vi "Create True Constant.vi"(5 "Sink":refnum<vi>, 6 "relative position/next to refnum":T1, 8 "error in (no error)":errorcluster, 11 "Diagram":refnum<vi>) -> (0 "error out":errorcluster, 2 "Output Terminal":refnum<vi>, 3 "constant out":refnum<vi>)   [LabVIEW 2018, in "Scripting Tools.lvlib"]
uses:
  Scripting Tools.lvlib
  <vilib>/Utility/miscctls.llb/LVPointTypeDef.ctl
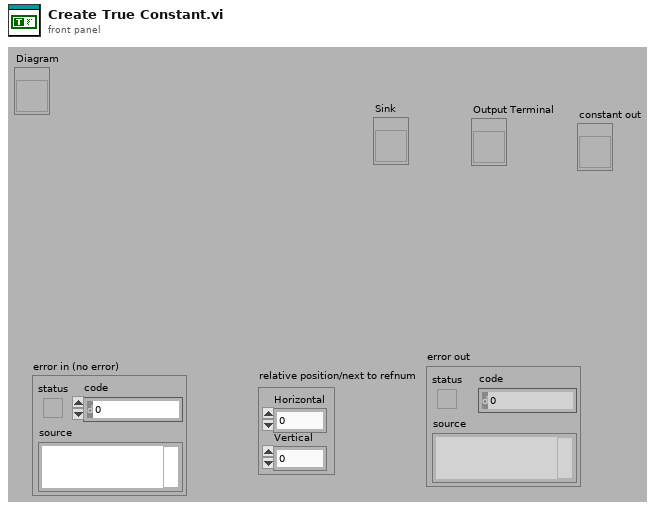
[diagram p1: front panel]
types:
  T1 = typedef "LVPointTypeDef.ctl" = cluster{"Horizontal":i16, "Vertical":i16}
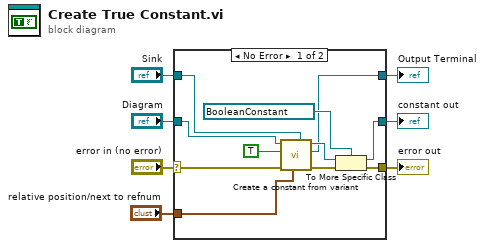
[diagram p0: block diagram]
diagram:
  n1 = case shown="No Error" "error in (no error)" {
    selector: "error in (no error)" -> [w16 w19]
    tunnel: "Diagram" -> [w18 _]
    tunnel: [w12 w19] -> w7
    tunnel: [w8 _] -> w6
    tunnel: [w9 _] -> w5
    tunnel: "relative position/next to refnum" -> [w17 _]
    tunnel: "Sink" -> [w15 _]
    frame No Error {
      n2 = call "Create a constant from variant.vi"("Terminal Sink"=w15, "relative position/next to refnum"=w17, "error in (no error)"=w16, "Constant Data"=TRUE, "Diagram"=w18) -> ("error out"=w13:errorcluster, "Terminal"=w8:refnum<vi>, "Const Refnum"=w10:refnum<vi>)  [unwired: 4 out]
      n3 = To More Specific Class(target class=refnum<vi> refnum ("reference out"), reference=w10, error in=w13) -> (specific class reference=w9:refnum<vi>, error out=w12:errorcluster)
    }
    frame Error {
    }
  }
  "Output Terminal" <- w6
  "error out" <- w7
  "constant out" <- w5
